vi "Lezeti_Power_Monitor_06.vi"() -> ()   [LabVIEW 2012]
doc: "This example shows how to use autosetup and acquire a waveform on a single channel."
uses:
  <instrlib>/RIGOL DS1000 Series/Public/Data/Read (Single Waveform).vi
  <vilib>/measure/madcrms.llb/Basic Averaged DC-RMS for 1 Chan.vi
  <vilib>/measure/mascope.llb/Cycle Average and RMS 1 chan.vi
  <vilib>/Utility/file.llb/Write To Spreadsheet File (DBL).vi
  <instrlib>/RIGOL DS1000 Series/RIGOL DS1000 Series.lvlib
  <vilib>/measure/NI_MAPro.lvlib
panel:
  in  "Threshold Wattage":dbl
  in  "Event Threshold Output":path
  out "Elapsed Time (s)":dbl
  in  "Power Output File":path
  out "Average Power (Watts)":dbl
  out "Instant Power Waveform":waveform(dbl)(graph)
  in  "Current Channel":u16(ring) items=["Channel 1", "Channel 2", "Channel 3", "Channel 4"]
  in  "Timeout":u32=10000
  out "IRMS":dbl
  out "Current Waveform":waveform(dbl)(graph)
  out "VRMS":dbl
  in  "Voltage Channel":u16(ring) items=["Channel 1", "Channel 2", "Channel 3", "Channel 4"]
  in  "Stop":bool
  in  "Timeout":u32=10000
  out "Voltage Waveform":waveform(dbl)(graph)
  in  "VISA resource name":refnum<visa-resource-name>
  # "For Lezeti Air Conditioning System (Greenpath Tech)\nBy Matsu Thornton\nJuly 2016"
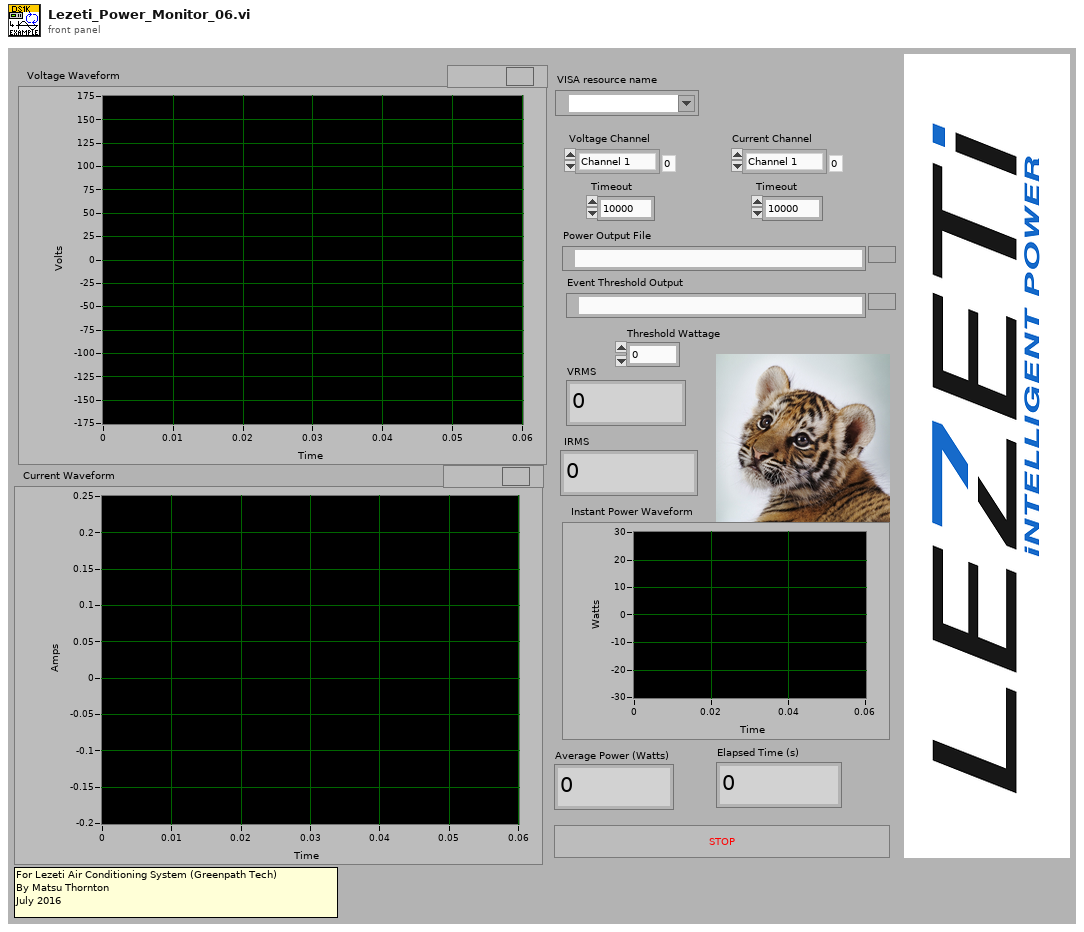
[diagram p1: front panel]
types:
  T1 = typedef "NI_Matrix.lvlib/RealMatrix.ctl" = dbl[][]
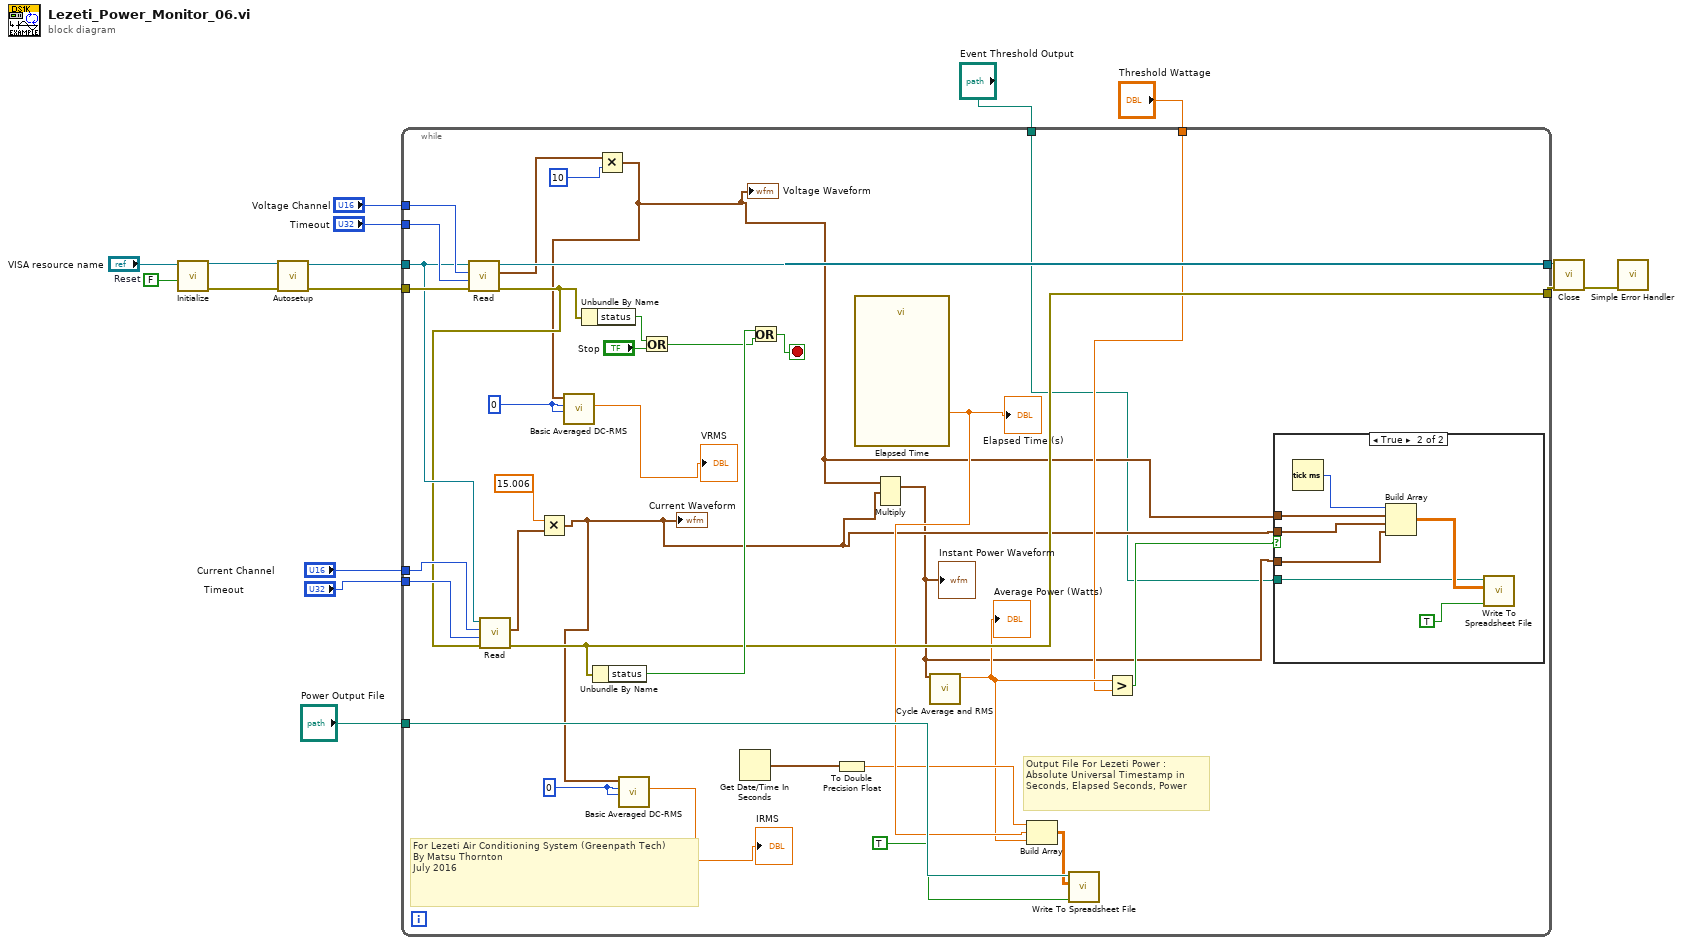
[diagram p0: block diagram]
diagram:
  w7 = FALSE  # Reset
  # "Output File For Lezeti Power :\nAbsolute Universal Timestamp in Seconds, Elapsed Seconds, Power"
  n1 = call <instrlib>:"Initialize.vi"("Reset (True)"=w7, "VISA resource name"="VISA resource name") -> ("error out"=w12:errorcluster, "VISA resource name out"=w11:refnum<visa-resource-name>)  [unwired: 2 in, 6 out]
  n2 = call <instrlib>:"Autosetup.vi"("error in (no error)"=w12, "VISA resource name"=w11) -> ("error out"=w9:errorcluster, "VISA resource name out"=w10:refnum<visa-resource-name>)  [unwired: 8 out]
  n3 = while {
    tunnel: w10 -> [w40]
    tunnel: w9 -> [w51]
    tunnel: [w50] -> w15
    tunnel: "Timeout" -> [w46]
    tunnel: "Voltage Channel" -> [w47]
    tunnel: "Current Channel" -> [w42]
    tunnel: "Timeout" -> [w41]
    tunnel: [w38] -> w4
    tunnel: "Power Output File" -> [w29]
    tunnel: "Event Threshold Output" -> [w17]
    tunnel: "Threshold Wattage" -> [w22]
    stop <- w30 stop-if-true
    w43 = 0
    w45 = 0
    # "For Lezeti Air Conditioning System (Greenpath Tech)\nBy Matsu Thornton\nJuly 2016"
    n4 = call-poly <instrlib>:"Read.vi"("error in (no error)"=w51, "Timeout (10000 ms)"=w46, "Channel (0: Channel 1)"=w47, "VISA resource name"=w40) -> ("error out"=w39:errorcluster, "Waveform Data"=w36:waveform(dbl), "VISA resource name out"=w50:refnum<visa-resource-name>)  [unwired: 5 out]
    n5 = call-poly <instrlib>:"Read.vi"("error in (no error)"=w39, "Timeout (10000 ms)"=w41, "Channel (0: Channel 1)"=w42, "VISA resource name"=w40) -> ("error out"=w38:errorcluster, "Waveform Data"=w34:waveform(dbl))  [unwired: 6 out]
    n6 = Multiply(x=15.006, y=w34) -> (x*y=w20:waveform(dbl))
    "Current Waveform" <- w20
    n7 = Unbundle By Name(w39) -> ("status"=w49:bool)
    n8 = Unbundle By Name(w38) -> ("status"=w44:bool)
    n9 = Multiply(x=w36, y=10) -> (x*y=w21:waveform(dbl))
    "Voltage Waveform" <- w21
    n10 = call-poly <vilib>:"Basic Averaged DC-RMS.vi"("window"=w45, "averaging type"=w45, "signal in"=w21) -> ("RMS value"=→"VRMS":dbl)  [unwired: 5 in, 3 out]
    n11 = call-poly <vilib>:"Basic Averaged DC-RMS.vi"("window"=w43, "averaging type"=w43, "signal in"=w20) -> ("RMS value"=→"IRMS":dbl)  [unwired: 5 in, 3 out]
    n12 = Or(x=w49, y="Stop") -> (x .or. y?=w31:bool)
    n13 = Get Date/Time In Seconds() -> (seconds since 1Jan1904=w26:timestamp)
    n14 = Or(x=w44, y=w31) -> (x .or. y?=w30:bool)
    n15 = To Double Precision Float(number=w26) -> (double precision float=w24:dbl)
    n16 = call "Elapsed Time"() -> ("Elapsed Time (s)"=w25:dbl)  [unwired: 12 in, 7 out]
    "Elapsed Time (s)" <- w25
    n17 = Multiply(1:w20, 2:w21) -> (0:w18:waveform(dbl))  [unwired: 1 in, 1 out]
    "Instant Power Waveform" <- w18
    n18 = call-poly <vilib>:"Cycle Average and RMS.vi"("signal in"=w18) -> ("cycle average"=w23:dbl)  [unwired: 7 in, 3 out]
    "Average Power (Watts)" <- w23
    n19 = Build Array(w24, w25, w23) -> (w27:T1)
    n20 = call-poly <vilib>:"Write To Spreadsheet File.vi"("append to file? (new file:F)"=TRUE, "2D data"=w27, "file path (dialog if empty)"=w29) -> ()  [unwired: 5 in, 1 out]
    n21 = Greater?(x=w23, y=w22) -> (0:w19:bool)
    n22 = case shown="True" w19 {
      tunnel: w21 -> [_ w57]
      tunnel: w20 -> [_ w56]
      tunnel: w18 -> [_ w55]
      tunnel: w17 -> [_ w52]
      frame False {
      }
      frame True {
        n23 = Tick Count (ms)() -> (millisecond timer value=w58:u32)
        n24 = Build Array(w58, w57, w56, w55) -> (w54:T1)
        n25 = call-poly <vilib>:"Write To Spreadsheet File.vi"("append to file? (new file:F)"=TRUE, "2D data"=w54, "file path (dialog if empty)"=w52) -> ()  [unwired: 5 in, 1 out]
      }
    }
  }
  n26 = call <instrlib>:"Close.vi"("error in (no error)"=w4, "VISA resource name"=w15) -> ("error out"=w16:errorcluster)  [unwired: 9 out]
  n27 = call <vilib>:"Simple Error Handler.vi"("error in (no error)"=w16) -> ()  [unwired: 1 in, 8 out]
